vi "SetPerioRegistration.vi"(8 "error in (no error)":errorcluster, 10 "Период регистрации":dbl, 11 "Archive in":refnum<class "Archive.lvclass">) -> (0 "error out":errorcluster, 3 "Archive out":refnum<class "Archive.lvclass">)   [LabVIEW 2010, in "Archive.lvclass"]
uses:
  Archive.lvclass
  Archive.lvclass/Archive.ctl
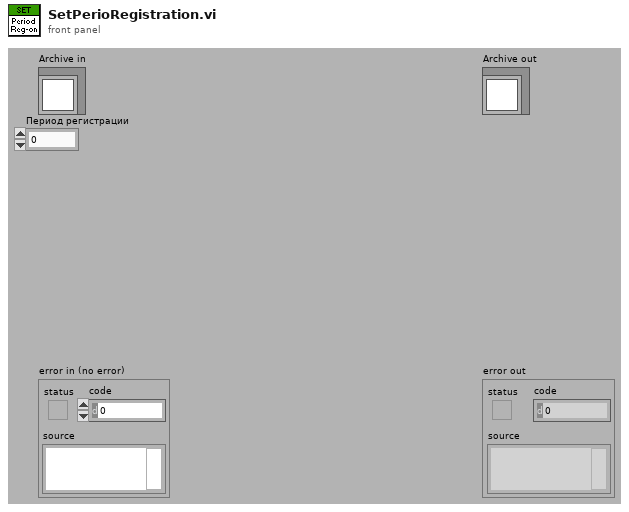
[diagram p1: front panel]
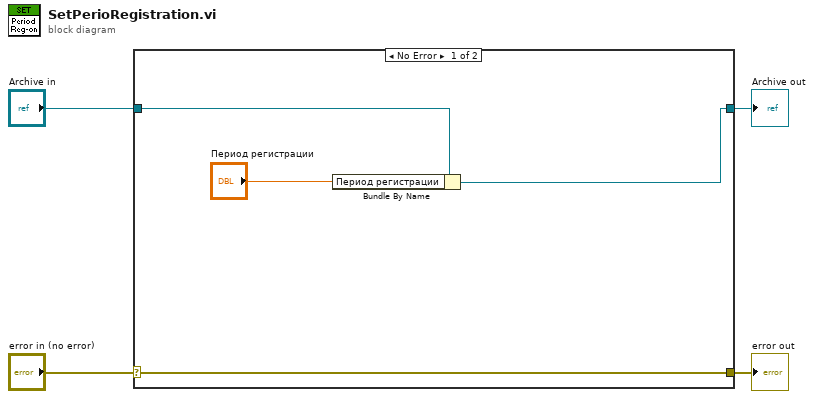
[diagram p0: block diagram]
diagram:
  n1 = case shown="No Error" "error in (no error)" {
    selector: "error in (no error)" -> [w8 w10]
    tunnel: [w8 w10] -> w3
    tunnel: [w6 w9] -> w1
    tunnel: "Archive in" -> [w7 w9]
    frame No Error {
      n2 = Bundle By Name(cluster=w7, "Период регистрации"="Период регистрации") -> (w6:refnum<class "Archive.lvclass">)
    }
    frame Error {
    }
  }
  "error out" <- w3
  "Archive out" <- w1
